vi "Write_Instr.vi"(8 "error in (no error)":errorcluster caption="entrée d'erreur (pas d'erreur)", 11 "Class Multimeter (Default) en entrée":refnum<class "Class Instrument Process.lvclass">) -> (0 "error out":errorcluster caption="sortie d'erreur", 3 "Class Multimeter (Default) en sortie":refnum<class "Class Instrument Process.lvclass">)   [LabVIEW 2020, in "Library Instrument & Equipement.lvlib" / "Library Instruments.lvlib" / "Class Instrument Process.lvclass"]
uses:
  Class Instrument Process.lvclass
  Class Instrument Process.lvclass/Class Instrument Process.ctl
  Instrument (Default)/Class Instrument (Default).lvclass
  Process/Process (Default)/Process (Default).lvclass
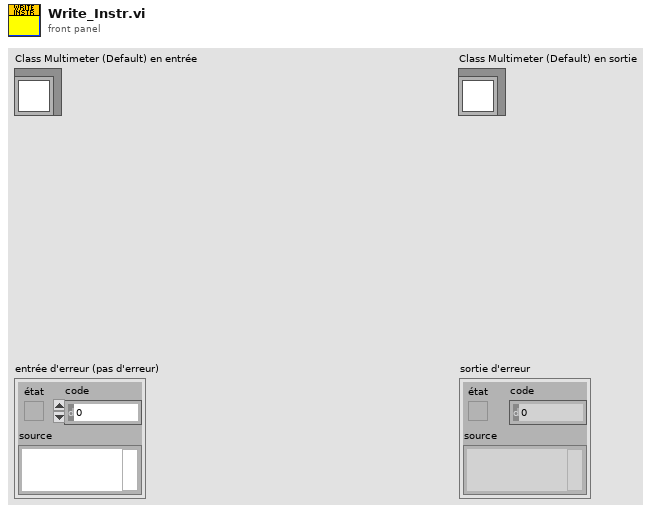
[diagram p1: front panel]
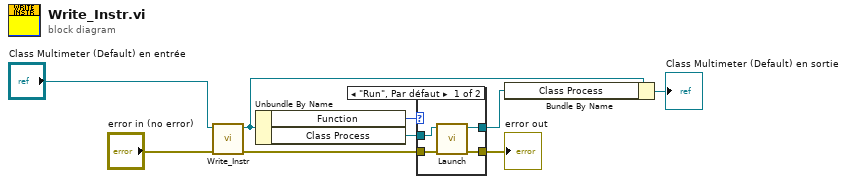
[diagram p0: block diagram]
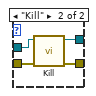
[diagram p2: hidden frame]
diagram:
  n1 = call-parent "Write_Instr.vi"("error in (no error)"="error in (no error)", "Class Multimeter (Default) en entrée"="Class Multimeter (Default) en entrée") -> ("error out"=w5:errorcluster, "Class Multimeter (Default) en sortie"=w3:refnum<class "Class Instrument Process.lvclass">)  [unwired: 8 in]
  n2 = Unbundle By Name(w3) -> ("Function"=w7:enum16{"Run", "Kill"}, "Class Process"=w6:refnum<class "Process (Default).lvclass">)
  n3 = case shown="\"Run\", Par défaut" w7 {
    tunnel: w6 -> [w13 w16]
    tunnel: w5 -> [w12 w17]
    tunnel: [w11 w14] -> w4
    tunnel: [w10 w15] -> w2
    frame "Run", Default {
      n4 = call-dynamic "Launch.vi"("error in (no error)"=w12, "Process (Default) en entrée"=w13) -> ("error out"=w11:errorcluster, "Process (Default) en sortie"=w10:refnum<class "Process (Default).lvclass">)  [unwired: 8 in]
    }
    frame "Kill" {
      n5 = call-dynamic "Kill.vi"("error in (no error)"=w17, "Process (Default) en entrée"=w16) -> ("error out"=w14:errorcluster, "Process (Default) en sortie"=w15:refnum<class "Process (Default).lvclass">)  [unwired: 8 in]
    }
  }
  "error out" <- w4
  n6 = Bundle By Name(cluster=w3, "Class Process"=w2) -> (→"Class Multimeter (Default) en sortie":refnum<class "Class Instrument Process.lvclass">)
